vi "RS_SMBV100A_QUERY.vi"(5 "milliseconds to wait":u32 max=60, 7 "String 2":string, 8 "error in":errorcluster {"code" format="%.0x"}, 9 "Session In":refnum<visa-resource-name>="COM3", 10 "InterfaceSettings In":T1, 11 "InterfaceType In":T3=enum."Prologix USB-GPIB") -> (0 "error out":errorcluster {"code" format="%.0x"}, 1 "Session Out":refnum<visa-resource-name>, 2 "InterfaceSettings Out":T1, 3 "InterfaceType Out":T3=enum."Prologix USB-GPIB", 4 "String":string)   [LabVIEW 2018]
uses:
  MOKO_LabViewLibrary/MokoLowLevel/MokoLowLovelControl/MLLC_InterfaceType.ctl
  MOKO_LabViewLibrary/MokoLowLevel/MokoLowLovelControl/MLLC_InterfaceSettings.ctl
  MOKO_LabViewLibrary/MokoLowLevel/MokoLowLovelControl/MLLC_InterfaceKind.ctl
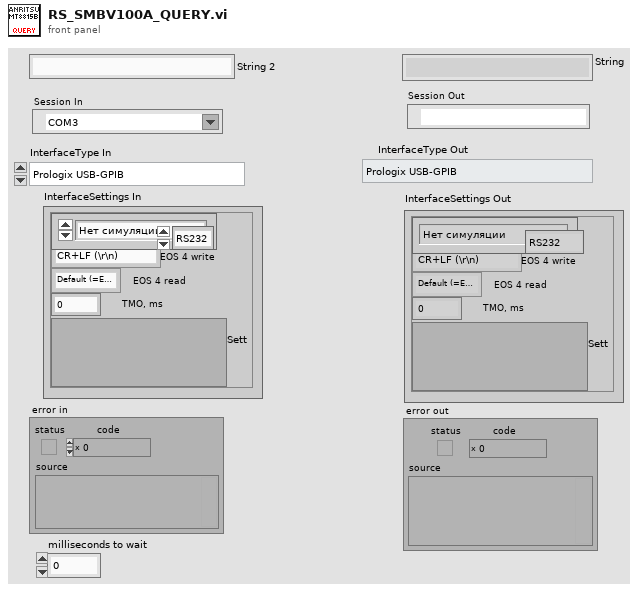
[diagram p1: front panel]
types:
  T1 = typedef "MLLC_InterfaceSettings.ctl" = cluster{"TMO, ms":i32, "EOS 4 write":enum16{"CR+LF (\\r\\n)", "CR (\\r)", "LF (\\n)", "None"}, "EOS 4 read":enum16{"Default (=EOS 4 write)", "CR (\\r)", "LF (\\n)", "None"}, "Sett":variant, "Simmulation":enum16{"Нет симуляции", "В ручную", "Игнорировать"}, "Interface?":T2}
  T2 = typedef "MLLC_InterfaceKind.ctl" = enum16{"RS232", "GPIB", "USB", "Ethernet", "another"}
  T3 = typedef "MLLC_InterfaceType.ctl" = enum16{"VISA", "Prologix USB-GPIB"}
  T4 = typedef "MLLC_Error.ctl" = errorcluster
  T5 = typedef "MLLC_ConnectCluster.ctl" = cluster{"InterfaceType":T3, "OpenedSession":T6, "InterfaceSettings":T7}
  T6 = typedef "MLLC_OpenedSession.ctl" = refnum<visa-resource-name>
  T7 = typedef "MLLC_InterfaceSettings.ctl" = cluster{"Interface":T2, "EOS 4 read":enum16{"Default (=EOS 4 write)", "CR (\\r)", "LF (\\n)", "None"}, "EOS 4 write":enum16{"CR+LF (\\r\\n)", "CR (\\r)", "LF (\\n)", "None"}, "TMO, ms":i32, "Sett":variant}
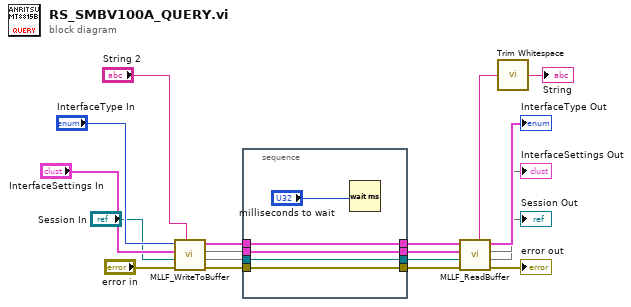
[diagram p0: block diagram]
diagram:
  n1 = call "MLLF_WriteToBuffer.vi"("String"="String 2", "error in"="error in", 7:"Session In", 8:"InterfaceSettings In", "DriverConnect in"="InterfaceType In") -> ("error out"=w3:T4, 1:w5, 2:w7, "DriverConnect out"=w9:T5)  [unwired: 1 in]
  n2 = stacked-sequence {
    tunnel: [w24] -> w10
    tunnel: w9 -> [w24]
    tunnel: [w23] -> w8
    tunnel: w7 -> [w23]
    tunnel: [w22] -> w6
    tunnel: w5 -> [w22]
    tunnel: [w21] -> w4
    tunnel: w3 -> [w21]
    frame #0 {
      n3 = Wait (ms)(milliseconds to wait="milliseconds to wait") -> ()  [unwired: 1 out]
    }
  }
  n4 = call "MLLF_ReadBuffer.vi"("Error In"=w4, 8:w6, 9:w8, "DriverConnect in"=w10) -> ("Error Out"=→"error out":errorcluster, 1:→"Session Out", 2:→"InterfaceSettings Out", "DriverConnect out"=→"InterfaceType Out":T5, "String"=w1:string)  [unwired: 2 in]
  n5 = call <vilib>:"Trim Whitespace.vi"("string"=w1) -> ("trimmed string"=→"String":string)  [unwired: 1 in]
